vi "applyWiringRules.vi"(8 "error in (no error)":errorcluster, 11 "PolymorphicInstance in":refnum<class "PolymorphicInstance.lvclass">) -> (0 "error out":errorcluster, 3 "PolymorphicInstance out":refnum<class "PolymorphicInstance.lvclass">)   [LabVIEW 2013, in "PolymorphicInstance.lvclass"]
uses:
  PolymorphicInstance.lvclass
  PolymorphicInstance.lvclass/PolymorphicInstance.ctl
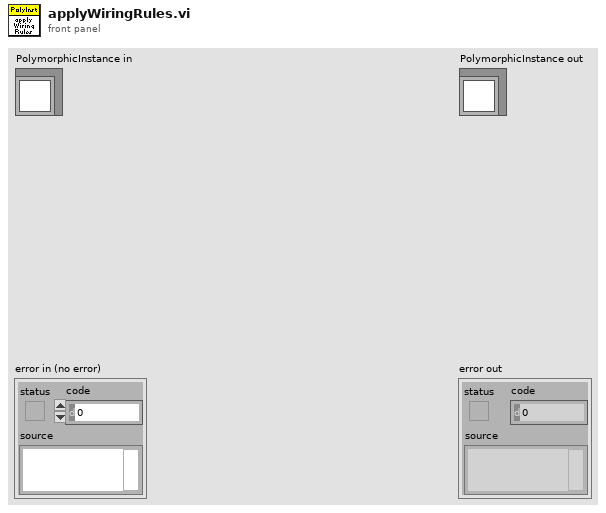
[diagram p1: front panel]
types:
  T1 = enum16{"Invalid Wire Rule", "Required", "Recommended", "Optional", "Dynamic Dispatch"}[]
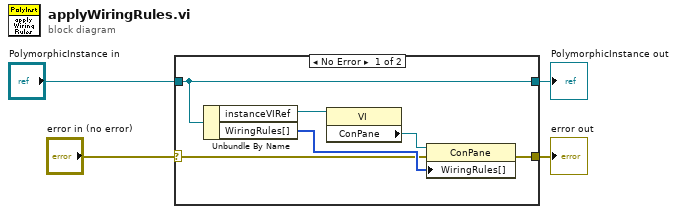
[diagram p0: block diagram]
diagram:
  n1 = case shown="No Error" "error in (no error)" {
    selector: "error in (no error)" -> [w6 w12]
    tunnel: [w5 w12] -> w3
    tunnel: [w10 w11] -> w1
    tunnel: "PolymorphicInstance in" -> [w10 w11]
    frame No Error {
      n2 = Unbundle By Name(w10) -> ("instanceVIRef"=w9:refnum<vi>, "WiringRules[]"=w7:T1)
      n3 = property class="VI"(reference=w9) -> ("ConPane"=w8:refnum<vi>)  [unwired: 1 in, 2 out]
      n4 = property class="ConPane"(reference=w8, error in=w6, "WiringRules[]"=w7) -> (error out=w5:errorcluster)  [unwired: 1 out]
    }
    frame Error {
    }
  }
  "error out" <- w3
  "PolymorphicInstance out" <- w1
